vi "word finder.vi"(9 "Pattern":string, 11 "String":string) -> (2 "finded?":bool)   [LabVIEW 2021]
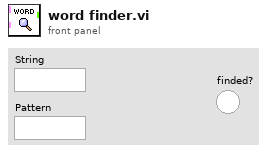
[diagram p1: front panel]
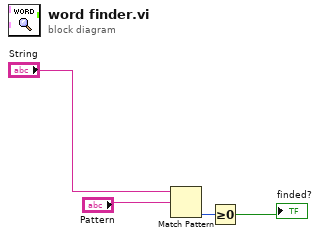
[diagram p0: block diagram]
diagram:
  n1 = Match Pattern(string="String", regular expression="Pattern") -> (offset past match=w4:i32)  [unwired: 1 in, 3 out]
  n2 = Greater Or Equal To 0?(x=w4) -> (x >= 0?=→"finded?":bool)
